vi "basic_settings.vi"(0 "VISA resource name":refnum<visa-resource-name>="TRIG", 1 "Burst enable?":bool, 2 "burst period (s)":dbl, 3 "burst count":i32, 5 "power level":string, 11 "error in (no error)":errorcluster) -> (4 "VISA resource name out":refnum<visa-resource-name>, 15 "error out":errorcluster)   [LabVIEW 2011]
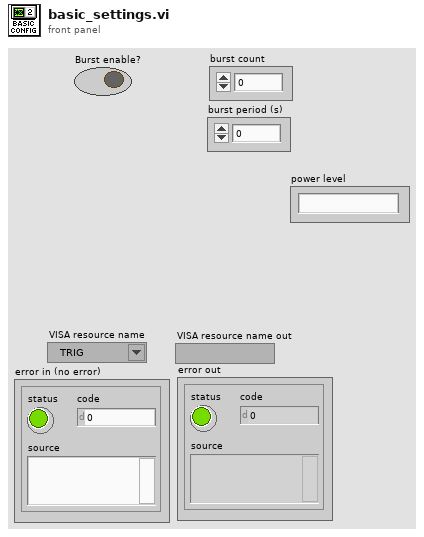
[diagram p1: front panel]
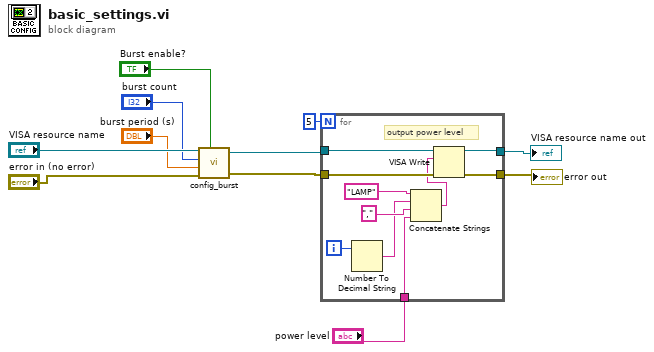
[diagram p0: block diagram]
diagram:
  n1 = call "config_burst.vi"("VISA resource name"="VISA resource name", "burst count"="burst count", "burst period (s)"="burst period (s)", "error in (no error)"="error in (no error)", "Burst enable?"="Burst enable?") -> ("VISA resource name out"=w4:refnum<visa-resource-name>, "error out"=w5:errorcluster)  [unwired: 1 in]
  n2 = for {
    N: 5 -> [_]
    tunnel: w4 -> [w20]
    tunnel: [w15] -> w11
    tunnel: w5 -> [w19]
    tunnel: [w18] -> w10
    tunnel: "power level" -> [w13]
    i -> [w12]
    # "output power level"
    n3 = Number To Decimal String(number=w12) -> (decimal integer string=w14:string)  [unwired: 1 in]
    n4 = Concatenate Strings("LAMP" ("Query 2"), w14, "," ("Query 2"), w13) -> (w16:string)
    n5 = VISA Write(VISA resource name=w20, write buffer=w16, error in (no error)=w19) -> (VISA resource name out=w15:refnum<visa-resource-name>, error out=w18:errorcluster)  [unwired: 1 out]
  }
  "VISA resource name out" <- w11
  "error out" <- w10
